vi "Toggle.vi"(3 "Trigger":bool, 12 "Initialize (F)":bool, 13 "Override to initialize value":bool) -> (23 "Output":bool)   [LabVIEW 2016]
doc: "The value of the Trigger terminal toggles the value of the output terminal. The starting value can be set by the initialize terminal. When the initialize terminal recives no value it is false.\n\nCreated by Team 4130 for use in the 2016-2017 FRC season"
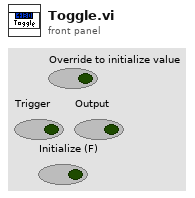
[diagram p1: front panel]
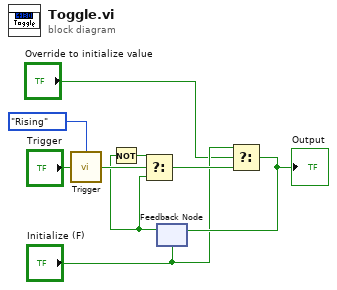
[diagram p0: block diagram]
diagram:
  n1 = call "Trigger.vi"("Enum"=enum16{"Falling", "Rising", "Both"}."Rising", "Button"="Trigger") -> ("Trigger"=w8:bool)  [unwired: 13 in]
  n2 = feedback #1("Initialize (F)") -> (w6:bool)
  n3 = Not(x=w6) -> (.not. x?=w7:bool)
  n4 = Select(t=w7, s=w8, f=w6) -> (s? t:f=w3:bool)
  n5 = Select(t="Initialize (F)", s="Override to initialize value", f=w3) -> (s? t:f=w4:bool)
  "Output" <- w4
  n6 = feedback-in #1(w4) -> ()
